vi "RunROSRIO_Master.vi"   [LabVIEW 2012]
uses:
  ROS/Code/_ROSDefinition.vi
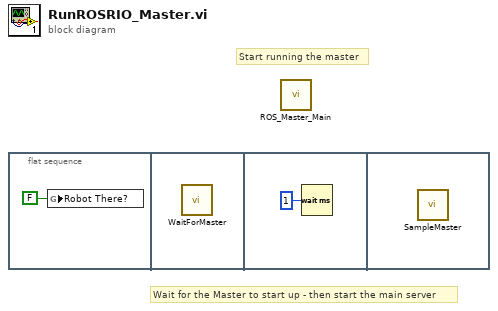
[diagram p0: block diagram]
diagram:
  # "Wait for the Master to start up - then start the main server"
  # "Start running the master"
  n1 = flat-sequence {
    frame #0 {
      n2 = global write "_ROSDefinition.vi" "Robot There?"(FALSE ("Robot There?")) -> ()
    }
    frame #1 {
      n3 = call "WaitForMaster.vi"() -> ()  [unwired: 1 in, 1 out]
    }
    frame #2 {
      n4 = Wait (ms)(milliseconds to wait=u32 1) -> ()  [unwired: 1 out]
    }
    frame #3 {
      n5 = call "SampleMaster.vi"() -> ()  [unwired: 12 in]
    }
  }
  n6 = call "ROS_Master_Main.vi"() -> ()  [unwired: 4 in]
